vi "Send and Receive.vi"() -> ()   [LabVIEW 2018]
uses:
  EPU452 Class/EPU452.lvclass
panel:
  in  "COM Port":refnum<visa-resource-name>="COM3"
  out "Response":string="help\r\nSystem Commands:\r\n help|?                                 This help\r\n version                                Get firmware version\r\n s|sample [hz]                          Sample at specified rate, 1Hz default\r\n get rates                              Get available sample rates\r\n i|interval <seconds>                   Interval sampling\r\n r                                      Take a single reading\r\n adc                                    Get raw ADC voltage values\r\n prompt <on|off>                        Enable or disable the command prompt\r\n get types                              Get a list of available function types\r\n set name                               Set device name <name>\r\n get name                               Get device name\r\n get serial                             Get device serial number\r\n set averaging <m>                      Set averaging period to <m> seconds (0.1\r\n                                        to 1.0)\r\n get averaging                          Get averaging period\r\n set channel <N> dp <n|auto>            Set the number of decimal places\r\n get channel <N> dp                     Get the number of decimal places\r\n get channel <N> function               Get the channel's current function\r\n get functions                          Show all channels' current functions\r\n set channel <N> function Off           Disable channel\r\n set channel <N> function Volt          Configure channel as Voltmeter\r\n set channel <N> function pH&ISE        Configure channel as pH/ISE\r\n set channel <N> function RTD           Configure channel as Pt 1k RTD\r\n set channel <N> function Therm         Configure channel as 10 k Thermistor\r\n set channel <N> function dO2           Configure channel as dO2\r\n set channel <N> function Bio           Configure channel as Biosensor\r\n set channel <N> function Cond          Configure channel as Conductivity\r\n\r\nChannel 1, 2, 3, 4: Voltmeter Commands:\r\n set channel <N> range <value>          Set input range (2000, 200)\r\n get channel <N> range                  Get input range\r\n get channel <N> ranges                 Get available ranges\r\n set channel <N> offset <0|off>         Remove any input offset\r\n set channel <N> offset auto            Automatically zero the input\r\n set channel <N> offset <m>             Set the offset to <m> mV\r\n get channel <N> offset                 Return the value of the zero offset\r\n\r\nNote that \"channel\" can be abbreviated to \"c\", \"ch\" or \"chan\".\r\n\r\nAdvanced Commands:\r\n get config                             Get system low-level configuration data\r\n start config                           Start low-level reconfiguration\r\n factoryreset                           Remove all configuration\r\nEPU452> "
  in  "Command":string="help"
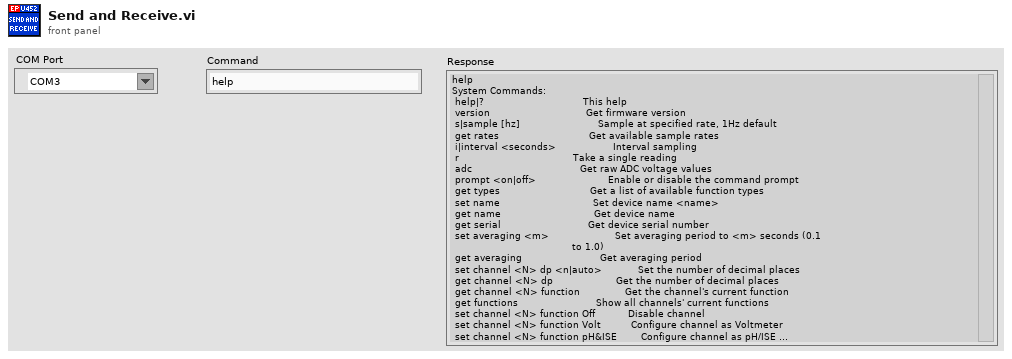
[diagram p1: front panel]
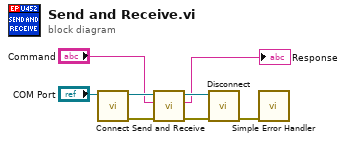
[diagram p0: block diagram]
diagram:
  n1 = call "Connect.vi"("COM Port"="COM Port") -> ("error out"=w3:errorcluster, "EPU452 out"=w2:refnum<class "EPU452.lvclass">)  [unwired: 9 in]
  n2 = call "Send and Receive.vi"("error in (no error)"=w3, "Command"="Command", "EPU452 in"=w2) -> ("error out"=w5:errorcluster, "Response"=→"Response":string, "EPU452 out"=w6:refnum<class "EPU452.lvclass">)  [unwired: 6 in]
  n3 = call "Disconnect.vi"("error in (no error)"=w5, "EPU452 in"=w6) -> ("error out"=w8:errorcluster)  [unwired: 9 in]
  n4 = call <vilib>:"Simple Error Handler.vi"("error in (no error)"=w8) -> ()  [unwired: 4 in, 5 out]
